vi "MoveToZero.vi"(9 "Decrease":dbl, 10 "Value":dbl) -> (2 "Out":dbl)   [LabVIEW 2017]
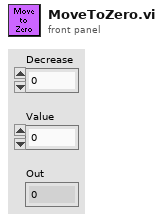
[diagram p1: front panel]
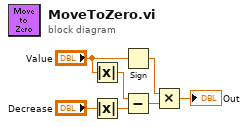
[diagram p0: block diagram]
diagram:
  n1 = Absolute Value(x="Value") -> (abs(x)=w4:dbl)
  n2 = Absolute Value(x="Decrease") -> (abs(x)=w1:dbl)
  n3 = Sign(1:"Value") -> (0:w5:dbl)
  n4 = Subtract(x=w4, y=w1) -> (x-y=w6:dbl)
  n5 = Multiply(x=w5, y=w6) -> (x*y=→"Out":dbl)
